vi "Set Rate (RPM).vi"(8 "error in (no error)":errorcluster, 10 "Rate (RPM)":dbl, 11 "Comp Motors with Brake in":refnum<class "Comp Motors with Brake.lvclass">) -> (0 "error out":errorcluster, 3 "Comp Motors with Brake out":refnum<class "Comp Motors with Brake.lvclass">)   [LabVIEW 2014, in "Comp Motors with Brake.lvlib" / "Comp Motors with Brake.lvclass"]
uses:
  Comp Motors with Brake.lvclass
  Comp Motors with Encoders/Comp Motors with Encoders Class/Comp Motors with Encoders.lvclass
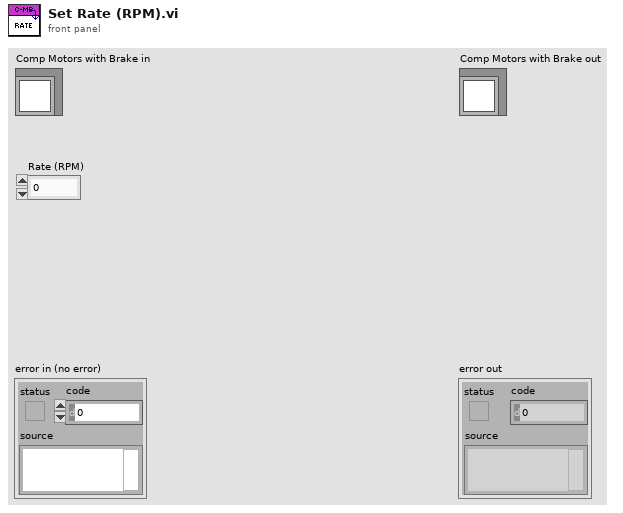
[diagram p1: front panel]
types:
  T1 = typedef "WPI_MotorControlDeviceRef.ctl" = cluster{"DeviceStatus":errorcluster, "Type":T2, "PWM":cluster{"Controller":T3, "PWM Channel":T4, "DeadBand":T5}, "CAN":cluster{"Device Number":u8, "Control Mode":T6, "Semaphore":T7, "Max Vout":dbl, "TalonSRX Control Mode":T8}, "Invert":bool, "TransformRef":T9, "InvTransformRef":T9}
  T2 = typedef "WPI_MotorControlType.ctl" = enum16{"PWM", "CAN", "CANTalonSRX"}
  T3 = typedef "FPGA_TypedefDigitalModule.ctl" = enum16{"Controller 1"}
  T4 = typedef "FPGA_DIOPWMChannel.ctl" = enum8{"PWM 0", "PWM 1", "PWM 2", "PWM 3", "PWM 4", "PWM 5", "PWM 6", "PWM 7", "PWM 8", "PWM 9", "PWM MXP 0", "PWM MXP 1", "PWM MXP 2", "PWM MXP 3", "PWM MXP 4", "PWM MXP 5", "PWM MXP 6", "PWM MXP 7", "PWM MXP 8", "PWM MXP 9", "Invalid"}
  T5 = typedef "WPI_PWMDeadband.ctl" = cluster{"Name":string, "maxPositivePwm":i32, "minPositivePwm":i32, "centerPwm":i32, "maxNegativePwm":i32, "minNegativePwm":i32, "angularRange":u16}
  T6 = typedef "WPI_CANJaguar_ControlMode.ctl" = enum8{"Percent VBus", "Current", "Speed", "Position", "Voltage"}
  T7 = typedef "Semaphore RefNum" = refnum<k1>
  T8 = typedef "WPI_CANTalonSRX_APIControlMode.ctl" = enum8{"Percent VBus", "Speed", "Position", "Slave", "Unchanged / Invalid"}
  T9 = typedef "WPI_PWMTransform_ConPane.ctl" = refnum<vi>
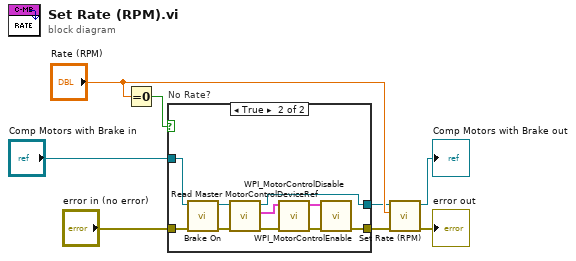
[diagram p0: block diagram]
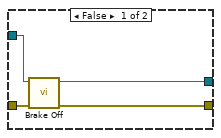
[diagram p2: hidden frame]
diagram:
  n1 = Equal To 0?(x="Rate (RPM)") -> (x = 0?=w6:bool)
  n2 = case "No Rate?" shown="True" w6 {
    tunnel: "Comp Motors with Brake in" -> [w12 w22]
    tunnel: "error in (no error)" -> [w10 w21]
    tunnel: [w11 w19] -> w2
    tunnel: [w9 w13] -> w1
    frame False {
      n3 = call-dynamic "Brake Off.vi"("error in (no error)"=w10, "Comp Motors with Brake in"=w12) -> ("error out"=w9:errorcluster, "Comp Motors with Brake out"=w11:refnum<class "Comp Motors with Brake.lvclass">)  [unwired: 8 in]
    }
    frame True {
      n4 = call-dynamic "Brake On.vi"("error in (no error)"=w21, "Comp Motors with Brake in"=w22) -> ("error out"=w16:errorcluster, "Comp Motors with Brake out"=w20:refnum<class "Comp Motors with Brake.lvclass">)  [unwired: 8 in]
      n5 = call-dynamic "Read Master MotorControlDeviceRef.vi"("error in (no error)"=w16, "Comp Motors with Encoders in"=w20) -> ("error out"=w15:errorcluster, "MotorControlDeviceRef"=w18:T1, "Comp Motors with Encoders out"=w19:refnum<class "Comp Motors with Brake.lvclass">)  [unwired: 7 in]
      n6 = call <vilib>:"WPI_MotorControlDisable.vi"("error in (no error)"=w15, "MotorControlDevRef"=w18) -> ("error out"=w14:errorcluster, "MotorControlDevRef"=w17:T1)  [unwired: 8 in]
      n7 = call <vilib>:"WPI_MotorControlEnable.vi"("error in (no error)"=w14, "CAN Jaguar Ref"=w17) -> ("error out"=w13:errorcluster)  [unwired: 8 in, 1 out]
    }
  }
  n8 = call-parent "Set Rate (RPM).vi"("error in (no error)"=w1, "Rate (RPM)"="Rate (RPM)", "Comp Motors with Encoders in"=w2) -> ("error out"=→"error out":errorcluster, "Comp Motors with Encoders out"=→"Comp Motors with Brake out":refnum<class "Comp Motors with Brake.lvclass">)  [unwired: 7 in]
